vi "Proceed.vi"(7 "component is ready (Y)":bool=TRUE, 8 "error in (no error)":errorcluster, 10 "ProceedMessage":refnum<class "ProceedMessage.lvclass">, 11 "TomoConversion in":refnum<class "TomoConversion.lvclass">) -> (0 "error out":errorcluster, 2 "all observers are ready?":bool, 3 "TomoConversion out":refnum<class "TomoConversion.lvclass">)   [LabVIEW 2012, in "TomoConversion.lvclass"]
uses:
  TomoConversion.lvclass
  <vilib>/Distrio/Murmex/ProceedMessage/ProceedMessage.lvclass
  TomoConversion.lvclass/TomoConversion.ctl
  <vilib>/Distrio/Murmex/Murmex/Murmex.lvclass
  <userlib>/_OpenG.lib/array/array.llb/Empty 1D Array (String)__ogtk.vi
panel:
  # "This method is called when the PROCEED\ntrigger is sent. \n\nOverride this method when your component needs to\nrespond to this trigger. \n\nCall parent for proper implementation"
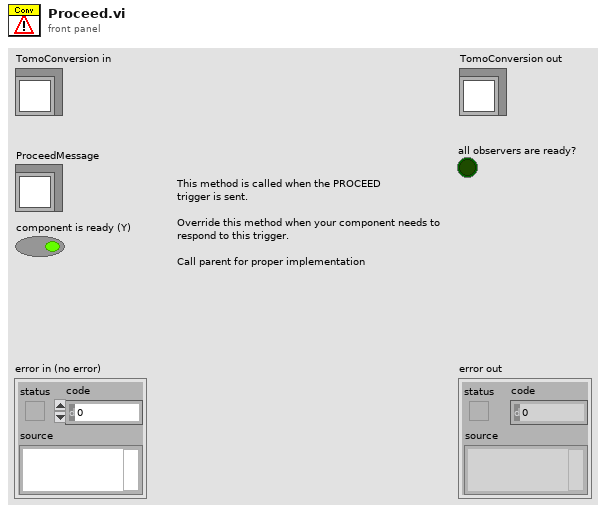
[diagram p1: front panel]
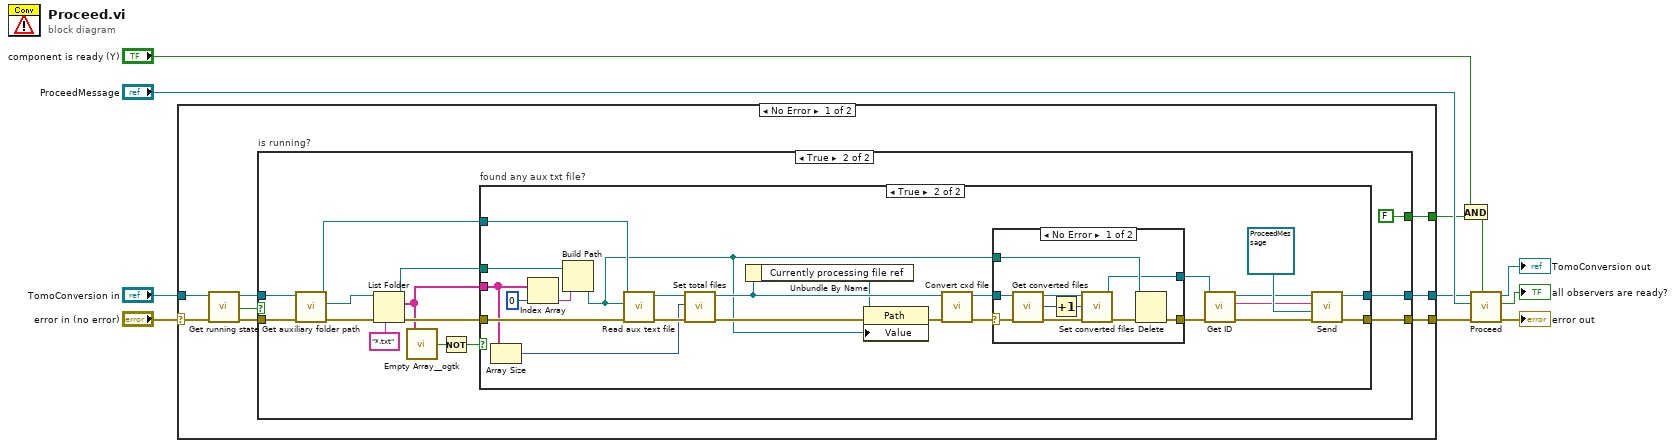
[diagram p0: block diagram]
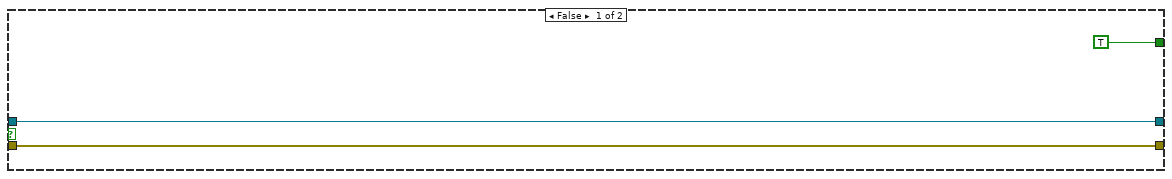
[diagram p2: hidden frame]
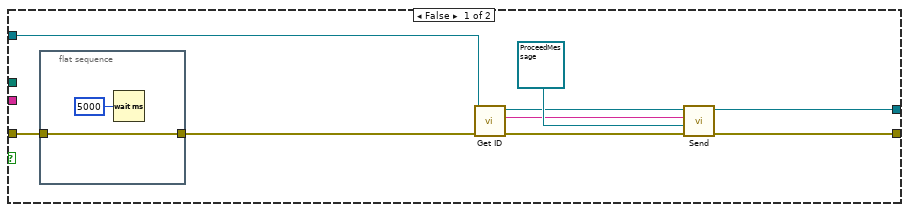
[diagram p3: hidden frame]
diagram:
  n1 = case shown="No Error" "error in (no error)" {
    selector: "error in (no error)" -> [w19 w85]
    tunnel: [w18 w85] -> w6
    tunnel: [w17 w84] -> w5
    tunnel: "TomoConversion in" -> [w15 w84]
    tunnel: [w12 _] -> w1
    frame No Error {
      n2 = call-dynamic "Get running state.vi"("error in (no error)"=w19, "TomoConversion in"=w15) -> ("error out"=w16:errorcluster, "is running?"=w13:bool, "TomoConversion out"=w14:refnum<class "TomoConversion.lvclass">)  [unwired: 7 in]
      n3 = case "is running?" shown="True" w13 {
        tunnel: [w21 w28] -> w18
        tunnel: [w22 w27] -> w17
        tunnel: w16 -> [w21 w26]
        tunnel: w14 -> [w22 w25]
        tunnel: [TRUE FALSE] -> w12
        frame False {
        }
        frame True {
          n4 = call-dynamic "Get auxiliary folder path.vi"("error in (no error)"=w26, "TomoConversion in"=w25) -> ("error out"=w35:errorcluster, "auxiliary folder path"=w34:path, "TomoConversion out"=w31:refnum<class "TomoConversion.lvclass">)  [unwired: 7 in]
          n5 = List Folder(path=w34, pattern="*.txt", error in=w35) -> (path out=w30:path, filenames=w29:string[], error out=w32:errorcluster)  [unwired: 1 in, 1 out]
          n6 = call-poly <userlib>:"Empty Array__ogtk.vi"("Array"=w29) -> ("Empty Array?"=w33:bool)  [unwired: 8 in]
          n7 = Not(x=w33) -> (.not. x?=w24:bool)
          n8 = case "found any aux txt file?" shown="True" w24 {
            tunnel: w32 -> [w39 w68]
            tunnel: w31 -> [w38 w67]
            tunnel: w30 -> [_ w70]
            tunnel: w29 -> [_ w54]
            tunnel: [w41 w60] -> w28
            tunnel: [w37 w59] -> w27
            frame False {
              n9 = flat-sequence {
                tunnel: [w47] -> w40
                tunnel: w39 -> [w47]
                frame #0 {
                  n10 = Wait (ms)(milliseconds to wait=u32 5000) -> ()  [unwired: 1 out]
                }
              }
              n11 = call <vilib>:"Get ID.vi"("error in (no error)"=w40, "Murmex in"=w38) -> ("error out"=w44:errorcluster, "component id"=w42:string, "Murmex out"=w43:refnum<class "TomoConversion.lvclass">)  [unwired: 7 in]
              n12 = call <vilib>:"Send.vi"("error in (no error)"=w44, "Message"=refnum<class "ProceedMessage.lvclass"> refnum ("Distrio Murmex 1.2:ProceedMessage"), "recipient"=w42, "Murmex in"=w43) -> ("error out"=w41:errorcluster, "Murmex out"=w37:refnum<class "TomoConversion.lvclass">)  [unwired: 6 in]
            }
            frame True {
              n13 = Array Size(array=w54) -> (size(s)=w53:i32)
              n14 = Index Array(array=w54, index=0) -> (element=w69:string)
              n15 = Build Path(base path=w70, name or relative path=w69) -> (appended path=w48:path)
              n16 = call-dynamic "Read aux text file.vi"("error in (no error)"=w68, "Aux text file path"=w48, "TomoConversion in"=w67) -> ("error out"=w56:errorcluster, "TomoConversion out"=w55:refnum<class "TomoConversion.lvclass">)  [unwired: 7 in]
              n17 = call-dynamic "Set total files.vi"("error in (no error)"=w56, "number of cxd files"=w53, "TomoConversion in"=w55) -> ("error out"=w50:errorcluster, "TomoConversion out"=w52:refnum<class "TomoConversion.lvclass">)  [unwired: 7 in]
              n18 = Unbundle By Name(w52) -> ("Currently processing file ref"=w51:refnum<vi>)
              n19 = property class="Path"(reference=w51, error in=w50, "Value"=w48) -> (error out=w49:errorcluster)  [unwired: 1 out]
              n20 = call-dynamic "Convert cxd file.vi"("error in (no error)"=w49, "TomoConversion in"=w52) -> ("error out"=w66:errorcluster, "TomoConversion out"=w58:refnum<class "TomoConversion.lvclass">)  [unwired: 8 in]
              n21 = case shown="No Error" w66 {
                selector: w66 -> [w81 w83]
                tunnel: w48 -> [w80 _]
                tunnel: [w79 w83] -> w64
                tunnel: w58 -> [w76 w82]
                tunnel: [w72 w82] -> w57
                frame No Error {
                  n22 = call-dynamic "Get converted files.vi"("error in (no error)"=w81, "TomoConversion in"=w76) -> ("error out"=w78:errorcluster, "converted cxd files"=w74:i32, "TomoConversion out"=w75:refnum<class "TomoConversion.lvclass">)  [unwired: 7 in]
                  n23 = Increment(x=w74) -> (x+1=w73:i32)
                  n24 = call-dynamic "Set converted files.vi"("error in (no error)"=w78, "converted cxd files"=w73, "TomoConversion in"=w75) -> ("error out"=w77:errorcluster, "TomoConversion out"=w72:refnum<class "TomoConversion.lvclass">)  [unwired: 7 in]
                  n25 = Delete(path (use dialog)=w80, error in=w77) -> (error out=w79:errorcluster)  [unwired: 3 in, 2 out]
                }
                frame Error {
                }
              }
              n26 = call <vilib>:"Get ID.vi"("error in (no error)"=w64, "Murmex in"=w57) -> ("error out"=w63:errorcluster, "component id"=w61:string, "Murmex out"=w62:refnum<class "TomoConversion.lvclass">)  [unwired: 7 in]
              n27 = call <vilib>:"Send.vi"("error in (no error)"=w63, "Message"=refnum<class "ProceedMessage.lvclass"> refnum ("Distrio Murmex 1.2:ProceedMessage"), "recipient"=w61, "Murmex in"=w62) -> ("error out"=w60:errorcluster, "Murmex out"=w59:refnum<class "TomoConversion.lvclass">)  [unwired: 6 in]
            }
          }
        }
      }
    }
    frame Error {
    }
  }
  n28 = And(x="component is ready (Y)", y=w1) -> (x .and. y?=w2:bool)
  n29 = call-parent "Proceed.vi"("component is ready (Y)"=w2, "error in (no error)"=w6, "ProceedMessage"="ProceedMessage", "Murmex in"=w5) -> ("error out"=→"error out":errorcluster, "all observers are ready?"=→"all observers are ready?":bool, "Murmex out"=→"TomoConversion out":refnum<class "TomoConversion.lvclass">)  [unwired: 5 in]
